vi "Parse Cluster.vi"(8 "error in":errorcluster, 11 "Cluster Refnum In":refnum<vi>) -> (0 "error out":errorcluster, 1 "Typedef?":bool, 2 "JSON ObjectSchema out":string, 3 "JSON Object Name":string, 4 "Typedef Name":string)   [LabVIEW 2020, in "JSON Schema Generator.lvlib"]
uses:
  JSON Schema Generator.lvlib
  <vilib>/JDP Science/JSONtext/LVClass Serializer/JSONtext LVClass Serializer.lvclass
  <vilib>/Utility/Data Type/NI_Data Type.lvlib
  Add Property (Numeric).vi
  <userlib>/_OpenG.lib/error/error.llb/openg_error.lvlib
  Add Property (Enum).vi
  Add Property (Array).vi
  Add Property (Cluster).vi
  9d05c4c8-8b14-4450-a203-34bc23169d95.vi
  <vilib>/JDP Science/JSONtext/JSONtext.lvlib
panel:
  # "e"
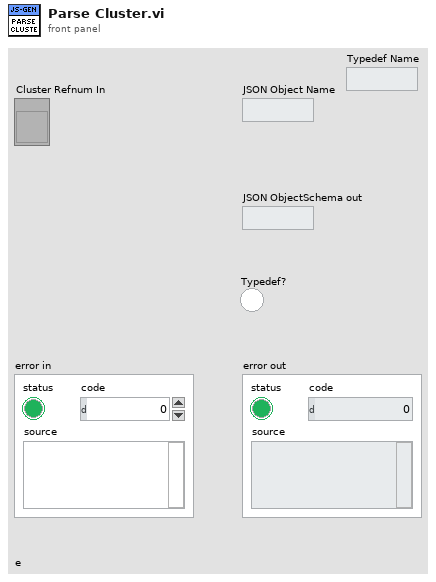
[diagram p1: front panel]
types:
  T1 = typedef "NI_Data Type.lvlib/Data Type.ctl" = enum8{"Invalid Type", "Void", "I8", "I16", "I32", "I64", "U8", "U16", "U32", "U64", "Single Float", "Double Float", "Extended Float", "Single Complex", "Double Complex", "Extended Complex", "Enum U8", "Enum U16", "Enum U32", "Enum U64", "Single Float With Unit", "Double Float With Unit", "Extended Float With Unit", "Single Complex with Unit", "Double Complex with Unit", "Extended Complex with Unit", "Boolean", "String", "Path", "Picture", "Tag", "Array", "Cluster", "Variant", "LV Variant", "Waveform", "Timestamp", "Digital Waveform", "Digital Data", "ExpressData", "Refnum", "External Data", "VI", "Poly VI", "LabVIEW Class Instance", "Fixed Point", "Set Collection", "Map Collection"}
  T2 = typedef "NI_Data Type.lvlib/Type Definition Info.ctl" = cluster{"Name":string, "Timestamp":u32}
  T3 = typedef "JSONtext.lvlib/JSON Value Type.ctl" = enum16{"Not a JSON Value", "JSON Object", "JSON Array", "String", "Number", "true", "false", "null"}
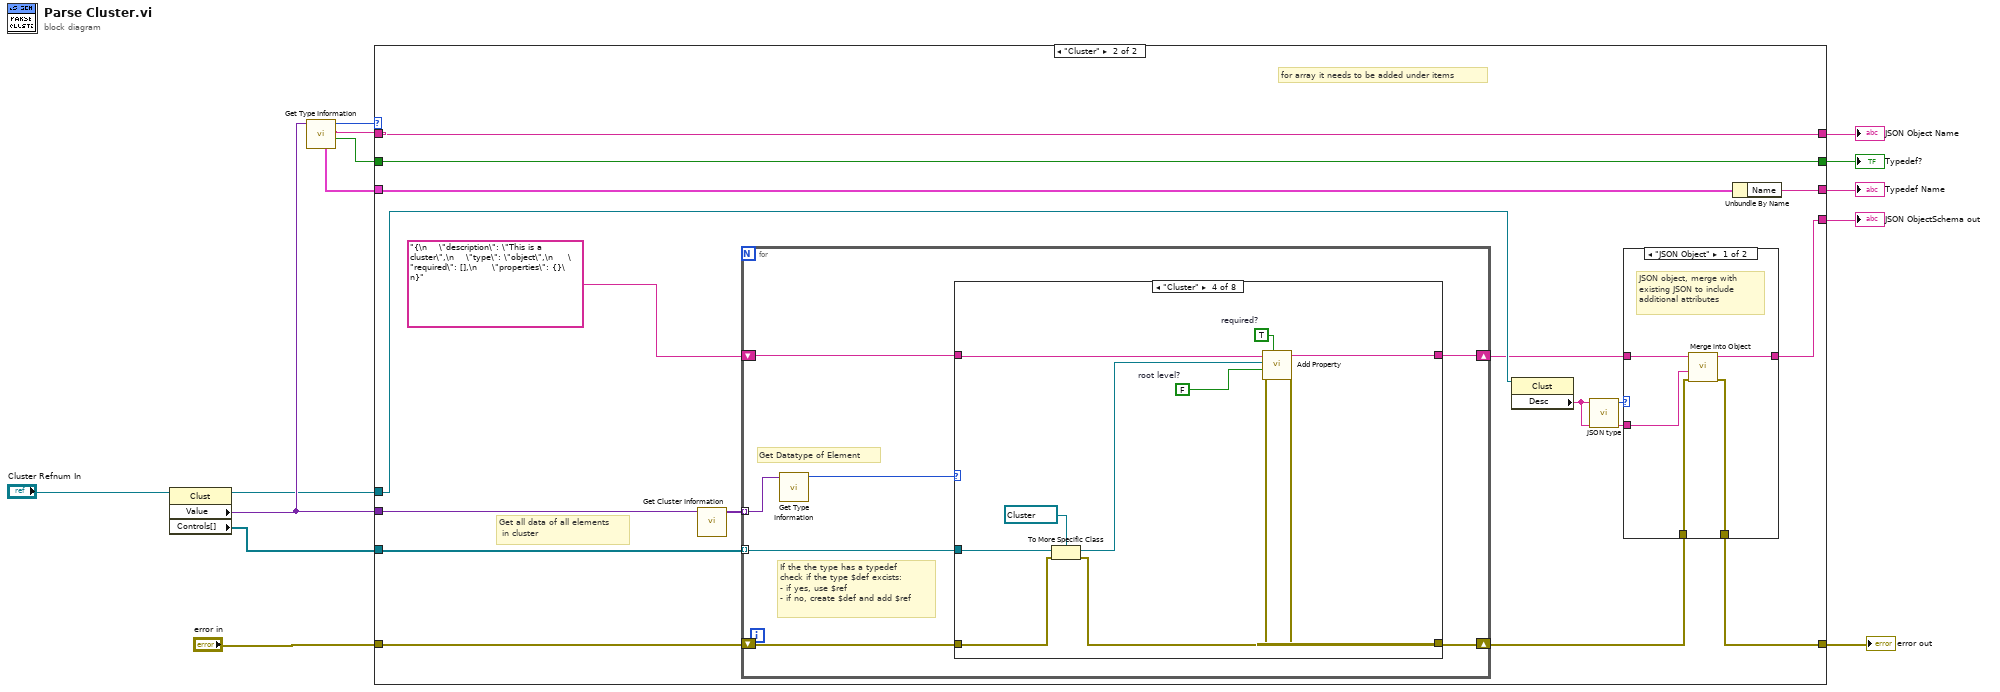
[diagram p0: block diagram]
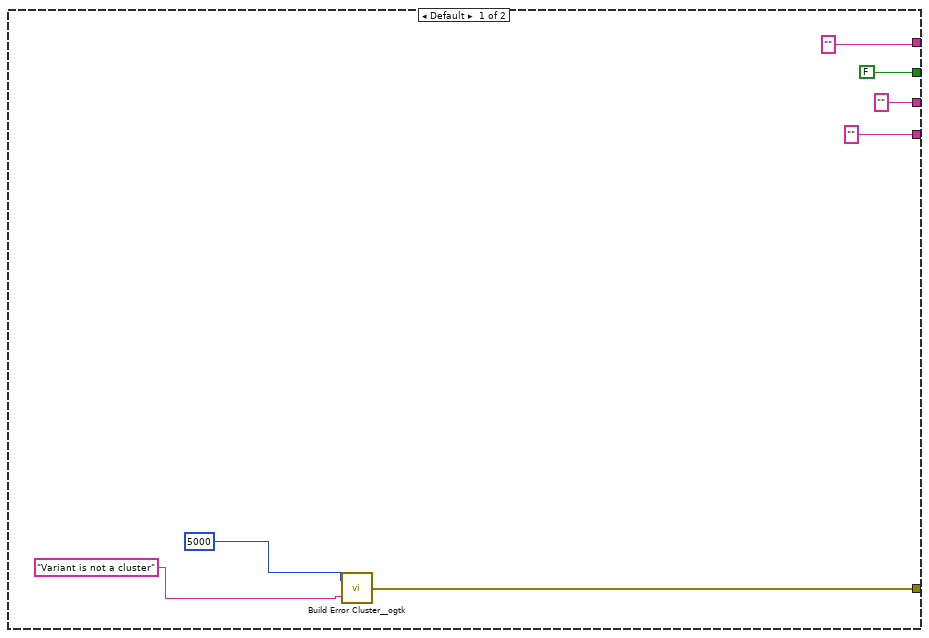
[diagram p2: hidden frame]
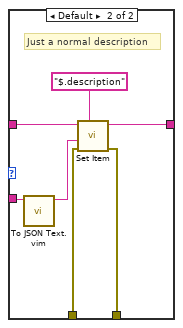
[diagram p3: hidden frame]
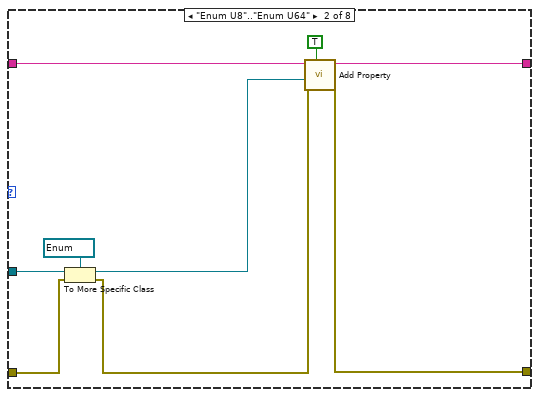
[diagram p5: hidden frame]
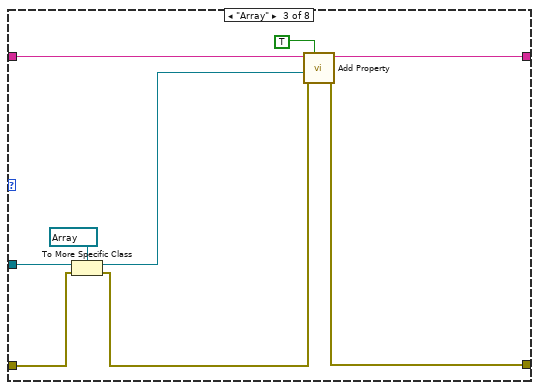
[diagram p6: hidden frame]
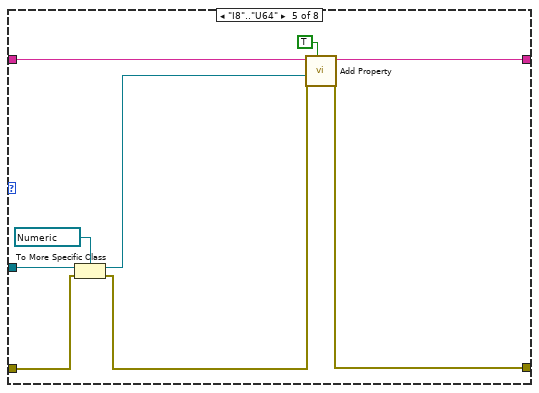
[diagram p7: hidden frame]
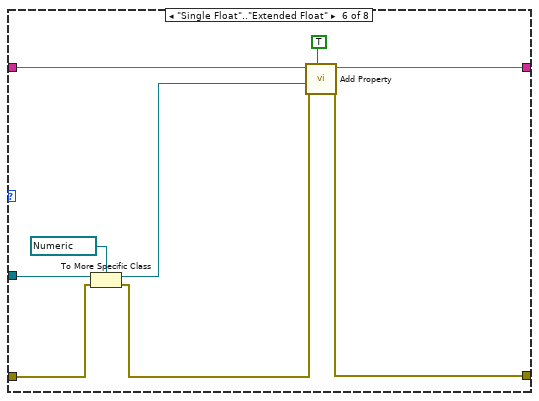
[diagram p8: hidden frame]
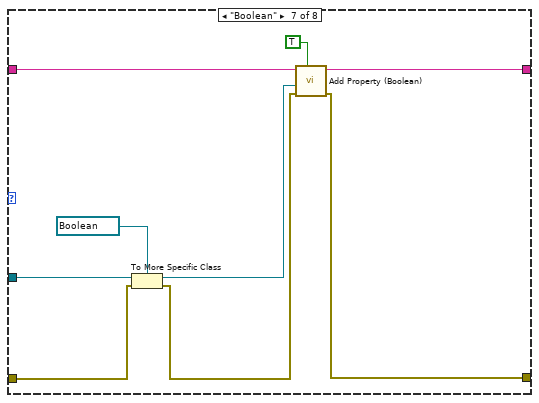
[diagram p9: hidden frame]
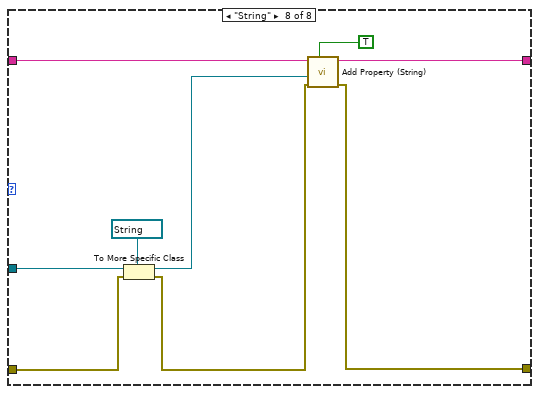
[diagram p10: hidden frame]
diagram:
  n1 = property on="Property Node" class="Clust"(reference="Cluster Refnum In") -> (reference out=w6:refnum<vi>, "Value"=w11:variant, "Controls[]"=w13:refnum<vi>[])  [unwired: 1 in, 1 out]
  n2 = call <vilib>:"Get Type Information.vi"("variant"=w11) -> ("type definition"=w4:bool, "name"=w10:string, "type"=w14:T1, "type definition info"=w3:T2)  [unwired: 6 in, 1 out]
  n3 = case shown="\"Cluster\"" w14 {
    tunnel: w11 -> [_ w37]
    tunnel: w13 -> [_ w35]
    tunnel: ["" ("<JSON>") w26] -> w9
    tunnel: w10 -> [_ w33]
    tunnel: [w19 w22] -> w8
    tunnel: "error in" -> [_ w34]
    tunnel: w6 -> [_ w28]
    tunnel: ["" ("name") w33] -> w5
    tunnel: w4 -> [_ w32]
    tunnel: w3 -> [_ w31]
    tunnel: [FALSE ("type definition") w32] -> w2
    tunnel: ["" ("Name") w30] -> w1
    frame Default {
      n4 = call <userlib>:"Build Error Cluster__ogtk.vi"("String to Prepend to source (\"\")"="Variant is not a cluster" ("String to Prepend to source (\"\")"), "code"=5000) -> ("error out"=w19:errorcluster)
    }
    frame "Cluster" {
      # "for array it needs to be added under items"
      # "Get all data of all elements\n in cluster"
      n5 = call <vilib>:"Get Cluster Information.vi"("variant"=w37) -> ("cluster elements"=w36:variant[])  [unwired: 9 in, 1 out]
      n6 = for {
        tunnel: w36 -> [w56] mode=indexing
        tunnel: w35 -> [w55] mode=indexing
        shift-right: [w53] -> w27
        shift-left: "{\n    \"description\": \"This is a cluster\",\n    \"type\": \"object\",\n     \"required\": [],\n     \"properties\": {}\n}" -> [w54]
        shift-right: [w52] -> w23
        shift-left: w34 -> [w51]
        # "If the the type has a typedef\ncheck if the type $def excists: \n- if yes, use $ref\n- if no, create $def and add $ref"
        # "Get Datatype of Element"
        n7 = call <vilib>:"Get Type Information.vi"("variant"=w56) -> ("type"=w50:T1)  [unwired: 6 in, 4 out]
        n8 = case shown="\"Cluster\"" w50 {
          tunnel: w55 -> [_ w67 w71 w85 w95 w99 w110 w119]
          tunnel: w54 -> [w58 w65 w76 w82 w91 w101 w112 w121]
          tunnel: [w58 w63 w75 w83 w92 w103 w113 w120] -> w53
          tunnel: [w57 w64 w74 w84 w90 w102 w108 w118] -> w52
          tunnel: w51 -> [w57 w59 w69 w77 w87 w96 w105 w114]
          frame Default {
          }
          frame "Enum U8".."Enum U64" {
            n9 = To More Specific Class(target class=refnum<vi> refnum ("Other Refnum"), reference=w67, error in=w59) -> (specific class reference=w61:refnum<vi>, error out=w60:errorcluster)
            n10 = call-poly "Add Property.vi"("Required?"=TRUE, "error in (no error)"=w60, "Enum In"=w61, "JSON Schema in"=w65) -> ("error out"=w64:errorcluster, "JSON SChema out"=w63:string)  [unwired: 6 in]
          }
          frame "Array" {
            n11 = To More Specific Class(target class=refnum<vi> refnum ("Other Refnum"), reference=w71, error in=w69) -> (specific class reference=w68:refnum<vi>, error out=w70:errorcluster)
            n12 = call-poly "Add Property.vi"("Required?"=TRUE, "error in (no error)"=w70, "Array Ref in"=w68, "JSON Schema in"=w76) -> ("error out"=w74:errorcluster, "JSON SChema out"=w75:string)  [unwired: 6 in]
          }
          frame "Cluster" {
            w79 = FALSE  # root level?
            w80 = TRUE  # required?
            n13 = To More Specific Class(target class=refnum<vi> refnum ("Other Refnum"), reference=w85, error in=w77) -> (specific class reference=w81:refnum<vi>, error out=w78:errorcluster)
            n14 = call-poly "Add Property.vi"("required?"=w80, "error in (no error)"=w78, "root level? (false)"=w79, "Cluster in"=w81, "JSON Schema in"=w82) -> ("error out"=w84:errorcluster, "JSON Schema out"=w83:string)  [unwired: 5 in]
          }
          frame "I8".."U64" {
            n15 = To More Specific Class(target class=refnum<vi> refnum ("Other Refnum"), reference=w95, error in=w87) -> (specific class reference=w89:refnum<vi>, error out=w88:errorcluster)
            n16 = call-poly "Add Property.vi"("Required?"=TRUE, "error in (no error)"=w88, "Numeric In"=w89, "JSON Schema in"=w91) -> ("error out"=w90:errorcluster, "JSON SChema out"=w92:string)  [unwired: 6 in]
          }
          frame "Single Float".."Extended Float" {
            n17 = To More Specific Class(target class=refnum<vi> refnum ("Other Refnum"), reference=w99, error in=w96) -> (specific class reference=w98:refnum<vi>, error out=w97:errorcluster)
            n18 = call-poly "Add Property.vi"("Required?"=TRUE, "error in (no error)"=w97, "Numeric In"=w98, "JSON Schema in"=w101) -> ("error out"=w102:errorcluster, "JSON SChema out"=w103:string)  [unwired: 6 in]
          }
          frame "Boolean" {
            n19 = To More Specific Class(target class=refnum<vi> refnum ("Other Refnum"), reference=w110, error in=w105) -> (specific class reference=w109:refnum<vi>, error out=w106:errorcluster)
            n20 = call "Add Property (Boolean).vi"("Required?"=TRUE, "error in (no error)"=w106, "String In"=w109, "JSON Schema in"=w112) -> ("error out"=w108:errorcluster, "JSON SChema out"=w113:string)  [unwired: 6 in]
          }
          frame "String" {
            n21 = To More Specific Class(target class=refnum<vi> refnum ("Other Refnum"), reference=w119, error in=w114) -> (specific class reference=w117:refnum<vi>, error out=w115:errorcluster)
            n22 = call "Add Property (String).vi"("Required?"=TRUE, "error in (no error)"=w115, "String In"=w117, "JSON Schema in"=w121) -> ("error out"=w118:errorcluster, "JSON SChema out"=w120:string)  [unwired: 6 in]
          }
        }
      }
      n23 = property class="Clust"(reference=w28) -> ("Desc"=w25:string)  [unwired: 1 in, 2 out]
      n24 = call <vilib>:"JSON type.vi"("JSON"=w25) -> ("JSON Value Type"=w24:T3)  [unwired: 9 in, 1 out]
      n25 = case shown="\"JSON Object\"" w24 {
        tunnel: w25 -> [w38 w49]
        tunnel: w27 -> [w42 w47]
        tunnel: [w41 w46] -> w26
        tunnel: w23 -> [w40 w44]
        tunnel: [w39 w43] -> w22
        frame "JSON Object" {
          # "JSON object, merge with \nexisting JSON to include\nadditional attributes"
          n26 = call <vilib>:"Merge into Object.vi"("error in (no error)"=w40, "JSON Object to Merge"=w38, "JSON"=w42) -> ("error out"=w39:errorcluster, "<JSON>"=w41:string)  [unwired: 6 in]
        }
        frame Default {
          # "Just a normal description"
          n27 = call "To JSON Text.vim"("Anything"=w49) -> ("<JSON>"=w45:string)  [unwired: 9 in, 1 out]
          n28 = call <vilib>:"Set Item.vi"("$Path or Item Name"="$.description", "error in (no error)"=w44, "JSON to Insert"=w45, "JSON"=w47) -> ("error out"=w43:errorcluster, "<JSON>"=w46:string)  [unwired: 4 in, 1 out]
        }
      }
      n29 = Unbundle By Name(w31) -> ("Name"=w30:string)
    }
  }
  "JSON ObjectSchema out" <- w9
  "error out" <- w8
  "JSON Object Name" <- w5
  "Typedef?" <- w2
  "Typedef Name" <- w1
